vi "AnalyzeWithinUncertainty_SIMPLE (SubVI).vi"(5 "Uncertainty on mean x":dbl, 7 "Mean x":dbl, 8 "Numeric":i32, 9 "y uncertainties":dbl[](array[numeric]), 10 "y values":dbl[](array[numeric]), 11 "x values":dbl[](array[numeric])) -> (1 "Uncertainty on mean y":dbl, 2 "Mean of y uncertainties":dbl, 3 "Mean y":dbl)   [LabVIEW 2016]
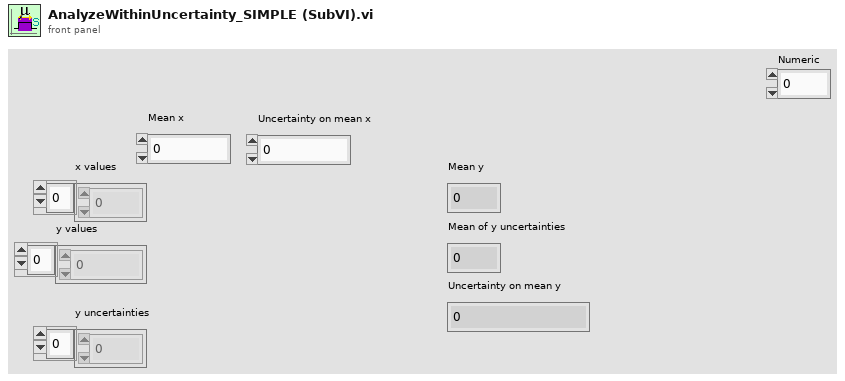
[diagram p1: front panel]
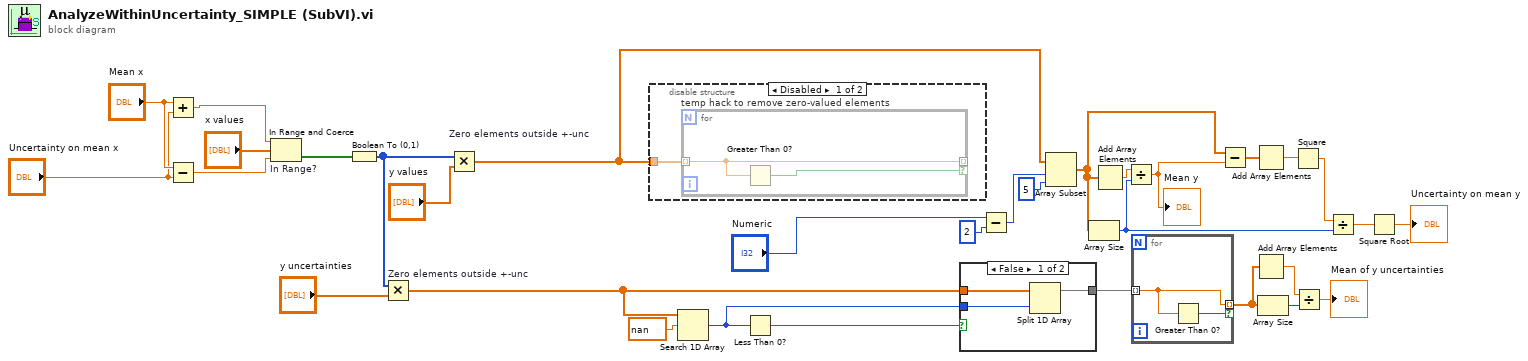
[diagram p0: block diagram]
diagram:
  n1 = Add(x="Mean x", y="Uncertainty on mean x") -> (x+y=w28:dbl)
  n2 = Subtract(x="Mean x", y="Uncertainty on mean x") -> (x-y=w27:dbl)
  n3 = In Range and Coerce "In Range?"(upper limit=w28, x="x values", lower limit=w27) -> (In Range?=w32:bool[])  [unwired: 1 out]
  n4 = Boolean To (0,1)(Boolean=w32) -> (0, 1=w25:i16[])
  n5 = Multiply "Zero elements outside +-unc"(x=w25, y="y uncertainties") -> (x*y=w12:dbl[])
  n6 = Multiply "Zero elements outside +-unc"(x=w25, y="y values") -> (x*y=w1:dbl[])
  n7 = disable-structure shown="Disabled" {
    disable-tunnel: w1 -> [w33 _]
    frame Disabled {
      n8 = for "temp hack to remove zero-valued elements" {
        tunnel: w33 -> [w35] mode=indexing
        tunnel: [w35] -> _ mode=indexing if=w34
        n9 = Greater Than 0?(x=w35) -> (x > 0?=w34:bool)
      }
    }
    frame Enabled {
    }
  }
  n10 = Search 1D Array(1D array=w12, element=nan) -> (index of element=w13:i32)  [unwired: 1 in]
  n11 = Less Than 0?(x=w13) -> (x < 0?=w14:bool)
  n12 = case shown="False" w14 {
    tunnel: w13 -> [w38 _]
    tunnel: w12 -> [w37 w39]
    tunnel: [w36 w39] -> w8
    frame False {
      n13 = Split 1D Array(array=w37, index=w38) -> (first subarray=w36:dbl[])  [unwired: 1 out]
    }
    frame True {
    }
  }
  n14 = Subtract(x="Numeric", y=2) -> (x-y=w4:i32)
  n15 = Array Subset(array=w1, index=w4, length=5) -> (w2:dbl[])
  n16 = Array Size(array=w2) -> (size(s)=w19:i32)
  n17 = Add Array Elements(numeric array=w2) -> (sum=w17:dbl)
  n18 = Divide(x=w17, y=w19) -> (x/y=w16:dbl)
  "Mean y" <- w16
  n19 = for {
    tunnel: w8 -> [w40] mode=indexing
    tunnel: [w40] -> w7 mode=indexing if=w41
    n20 = Greater Than 0?(x=w40) -> (x > 0?=w41:bool)
  }
  n21 = Subtract(x=w2, y=w16) -> (x-y=w18:dbl[])
  n22 = Add Array Elements(numeric array=w18) -> (sum=w20:dbl)
  n23 = Add Array Elements(numeric array=w7) -> (sum=w11:dbl)
  n24 = Array Size(array=w7) -> (size(s)=w10:i32)
  n25 = Square(x=w20) -> (x^2=w21:dbl)
  n26 = Divide(x=w11, y=w10) -> (x/y=→"Mean of y uncertainties":dbl)
  n27 = Divide(x=w21, y=w19) -> (x/y=w22:dbl)
  n28 = Square Root(x=w22) -> (sqrt(x)=→"Uncertainty on mean y":dbl)
